vi "Visual Map.vi"() -> ()   [LabVIEW 2017, in "Bubble.lvclass"]
uses:
  Bubble.lvclass
  Role Enum.ctl
  State Enum.ctl
panel:
  out "Array 7":u32[][](array[colorbox])=[[13816530, 13816530, 13816530, 13816530, 13816530, 13816530, 13816530], [3381759, 3381759, 3381759, 13816530, 13816530, 13816530, 13816530], [6618880, 6618880, 6618880, 13816530, 13816530, 13816530, 13816530]]
  out "Array 6":u32[][](array[colorbox])=[[13816530, 13816530, 3381759, 3381759, 13816530, 13816530, 13816530], [13816530, 13816530, 6618880, 6618880, 13816530, 13816530, 13816530], [3381759, 3381759, 13816530, 13816530, 13816530, 13816530, 13816530], [6618880, 6618880, 13816530, 13816530, 13816530, 13816530, 13816530]]
  out "Array 5":u32[][](array[colorbox])=[[13816530, 3381759, 3381759, 13816530, 3381759, 3381759, 13816530], [13816530, 6618880, 6618880, 13816530, 6618880, 6618880, 13816530], [13816530, 13816530, 13816530, 13816530, 13816530, 13816530, 13816530], [13816530, 3381759, 3381759, 13816530, 3381759, 3381759, 13816530], [13816530, 6618880, 6618880, 13816530, 6618880, 6618880, 13816530], [13816530, 13816530, 13816530, 13816530, 13816530, 13816530, 13816530]]
  in  "State":T1=enum."Empty Parent"
  in  "Role":T2
  out "Array 4":u32[][](array[colorbox])=[[13816530, 3381759, 13816530, 3381759], [13816530, 6618880, 13816530, 6618880], [3381759, 13816530, 3381759, 13816530], [6618880, 13816530, 6618880, 13816530], [13816530, 3381759, 13816530, 3381759], [13816530, 6618880, 13816530, 6618880]]
  # "Use View and Map to update surroundings\n\nUse Role and Map to decide action\n\nUpdate map with action"
  # "Parent\nChild\nMove\nWall\nOutside"
  # "Attacked\nOccupied\nEmpty Child\nEmpty Move\nOutside\nEmpty Parent\nEmpty Wall\nPop\nEnemy"
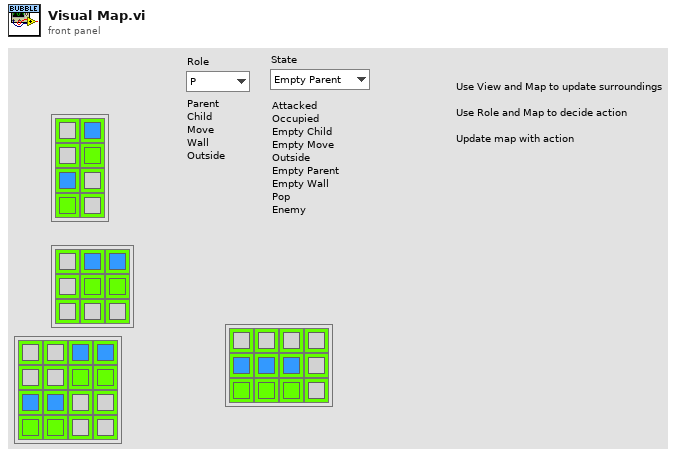
[diagram p1: front panel]
types:
  T1 = typedef "Bubble.lvclass/State Enum.ctl" = enum16{"Attacked", "Occupied", "Empty Child", "Empty Move", "Outside", "Empty Parent", "Empty Wall", "Enemy"}
  T2 = typedef "Bubble.lvclass/Role Enum.ctl" = enum16{"P", "C", "M", "W", "O"}
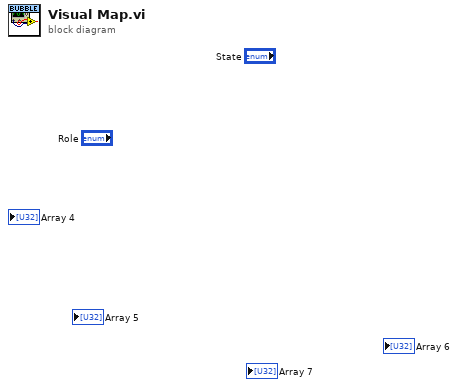
[diagram p0: block diagram]
diagram:
